vi "Benchmark.vi"() -> ()   [LabVIEW 2020, in "Test Method Finding Test.lvclass"]
uses:
  Test Method Finding Test.lvclass
  Test Doubles/Test Case Test Double/Test Case Test Double.lvclass
panel:
  in  "Implementation":enum16{"xml_lib", "string parsing"}(ring)
  out "Time [ms]":u32
  out "Array":path[](array[path])
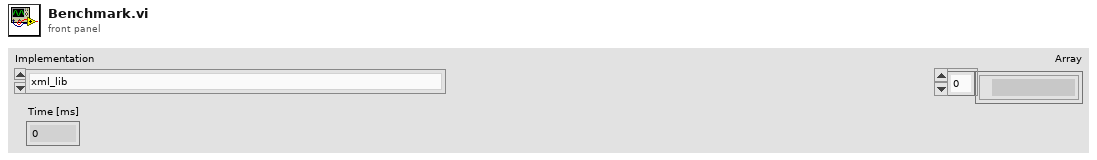
[diagram p1: front panel]
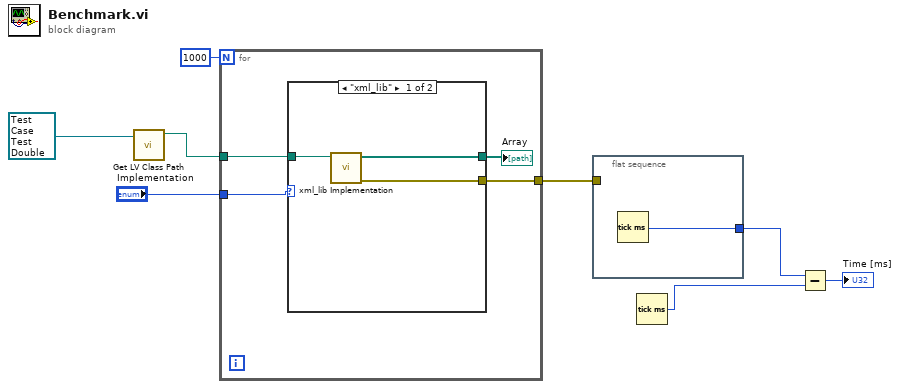
[diagram p0: block diagram]
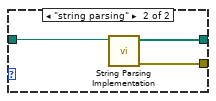
[diagram p2: hidden frame]
diagram:
  n1 = call <vilib>:"Get LV Class Path.vi"("object"=refnum<class "Test Case Test Double.lvclass"> refnum ("Test Case Test Double.lvclass")) -> ("class path"=w6:path)  [unwired: 9 in, 1 out]
  n2 = for {
    N: 1000 -> [_]
    tunnel: w6 -> [w12]
    tunnel: [w11] -> w5
    tunnel: "Implementation" -> [w10]
    n3 = case shown="\"xml_lib\"" w10 {
      tunnel: w12 -> [w15 w16]
      tunnel: [w14 w17] -> w11
      tunnel: [w13 w18] -> w9
      frame "xml_lib" {
        n4 = call "xml_lib Implementation.vi"("class path"=w15) -> ("error out"=w14:errorcluster, "Array"=w13:path[])  [unwired: 9 in]
      }
      frame "string parsing" {
        n5 = call "String Parsing Implementation.vi"("class path"=w16) -> ("error out"=w17:errorcluster, "Array"=w18:path[])  [unwired: 9 in]
      }
    }
    "Array" <- w9
  }
  n6 = flat-sequence {
    tunnel: w5 -> [_]
    tunnel: [w19] -> w4
    frame #0 {
      n7 = Tick Count (ms)() -> (millisecond timer value=w19:u32)
    }
  }
  n8 = Tick Count (ms)() -> (millisecond timer value=w3:u32)
  n9 = Subtract(x=w4, y=w3) -> (x-y=→"Time [ms]":u32)
